vi "Potenzac.vi"(3 "Npp_Frame":i32, 4 "I":dbl[](array[numeric]), 5 "V":dbl[](array[numeric])) -> (0 "Apparent Power":dbl, 1 "Reactive Power":dbl, 2 "Active Power":dbl)   [LabVIEW 2018]
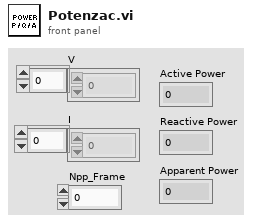
[diagram p1: front panel]
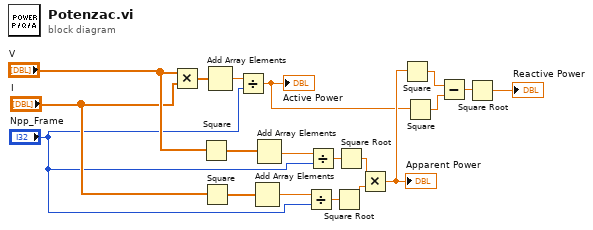
[diagram p0: block diagram]
diagram:
  n1 = Multiply(x="V", y="I") -> (x*y=w19:dbl[])
  n2 = Square(x="V") -> (x^2=w15:dbl[])
  n3 = Square(x="I") -> (x^2=w14:dbl[])
  n4 = Add Array Elements(numeric array=w19) -> (sum=w18:dbl)
  n5 = Divide(x=w18, y="Npp_Frame") -> (x/y=w6:dbl)
  "Active Power" <- w6
  n6 = Add Array Elements(numeric array=w14) -> (sum=w12:dbl)
  n7 = Add Array Elements(numeric array=w15) -> (sum=w13:dbl)
  n8 = Divide(x=w12, y="Npp_Frame") -> (x/y=w10:dbl)
  n9 = Divide(x=w13, y="Npp_Frame") -> (x/y=w11:dbl)
  n10 = Square Root(x=w10) -> (sqrt(x)=w8:dbl)
  n11 = Square Root(x=w11) -> (sqrt(x)=w9:dbl)
  n12 = Multiply(x=w9, y=w8) -> (x*y=w7:dbl)
  "Apparent Power" <- w7
  n13 = Square(x=w7) -> (x^2=w4:dbl)
  n14 = Square(x=w6) -> (x^2=w5:dbl)
  n15 = Subtract(x=w4, y=w5) -> (x-y=w3:dbl)
  n16 = Square Root(x=w3) -> (sqrt(x)=→"Reactive Power":dbl)
